vi "libssh2_userauth_password_ex.vi"(7 "passwd_change_cb":u64, 8 "error in (no error)":errorcluster, 9 "password":string, 10 "username":string, 11 "session":T1) -> (0 "error out":errorcluster)   [LabVIEW 2013, in "libssh2.lvlib"]
doc: "Authenticate a session using a password with a custom password change callback."
uses:
  libssh2.lvlib
  Session Refnum.ctl
  Not A Session.vi
  <vilib>/Utility/error.llb/Error Cluster From Error Code.vi
  Global Settings.vi
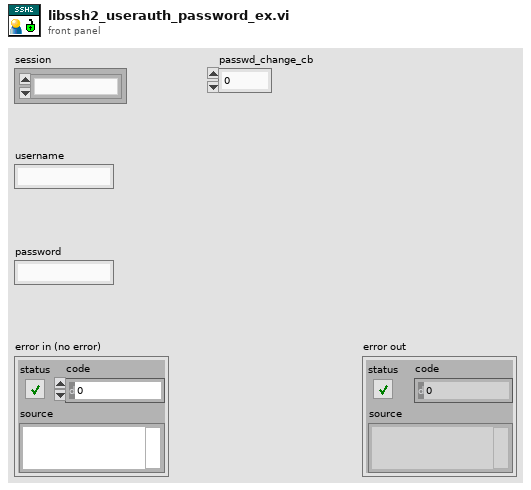
[diagram p1: front panel]
types:
  T1 = typedef "libssh2.lvlib/Session Refnum.ctl" = refnum<k1>
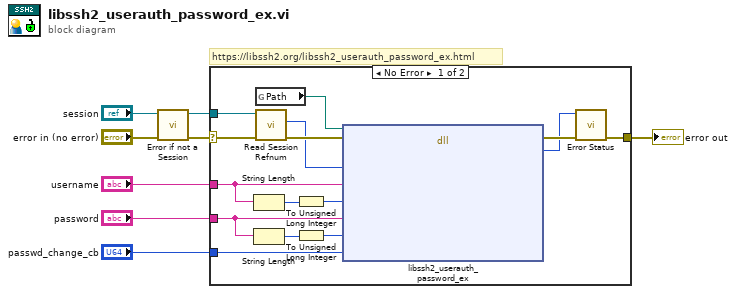
[diagram p0: block diagram]
diagram:
  # "https://libssh2.org/libssh2_userauth_password_ex.html"
  n1 = call "Error if not a Session.vi"("error in (no error)"="error in (no error)", "session"="session") -> ("error out"=w3:errorcluster, "session out"=w1:T1)  [unwired: 8 in]
  n2 = case shown="No Error" w3 {
    selector: w3 -> [w20 w24]
    tunnel: "username" -> [w23 _]
    tunnel: "password" -> [w22 _]
    tunnel: "passwd_change_cb" -> [w21 _]
    tunnel: [w19 w24] -> w5
    tunnel: w1 -> [w18 _]
    frame No Error {
      n3 = String Length(string=w23) -> (length=w13:i32)
      n4 = String Length(string=w22) -> (length=w14:i32)
      n5 = global read "Global Settings.vi" "Path"() -> (w10:path)
      n6 = call "Read Session Refnum.vi"("error in (no error)"=w20, "session"=w18) -> ("error out"=w12:errorcluster, "LIBSSH2_SESSION*"=w11:u64)  [unwired: 5 in, 3 out]
      n7 = To Unsigned Long Integer(number=w13) -> (unsigned 32bit integer=w17:u32)
      n8 = To Unsigned Long Integer(number=w14) -> (unsigned 32bit integer=w16:u32)
      n9 = dll-call lib="?" fn="libssh2_userauth_password_ex"(path in=w10, error in=w12, "session"=w11, "username"=w23, "username_len"=w17, "password"=w22, "password_len"=w16, "passwd_change_cb"=w21) -> (error out=w15:errorcluster, "return value"=w9:i32)  [unwired: 7 in, 1 out]
      n10 = call "Error Status.vi"("error in (no error)"=w15, "return value"=w9) -> ("error out"=w19:errorcluster)  [unwired: 8 in, 1 out]
    }
    frame Error {
    }
  }
  "error out" <- w5
